vi "XY Graph Remove Head Outliers.vi"(8 "Error In":errorcluster, 9 "Peak Index (-1: unknown)":i32=-1, 11 "Plot in":cluster{"t Array":dbl[], "Array":dbl[]}) -> (0 "Error Out":errorcluster, 1 "# Outliers":i32, 3 "Plot out":cluster{"t Array":dbl[], "Array":dbl[]})   [LabVIEW 2021, in "XY Graph Add-Ons.lvlib"]
uses:
  XY Graph Add-Ons.lvlib
  <vilib>/gmath/statdist.llb/Normal Random.vi
  <vilib>/Analysis/NI_AALBase.lvlib
  <vilib>/gmath/NI_Gmath.lvlib
panel:
  # "see the License on the block diagram (Ctrl+E or Window:Show Block Diagram)"
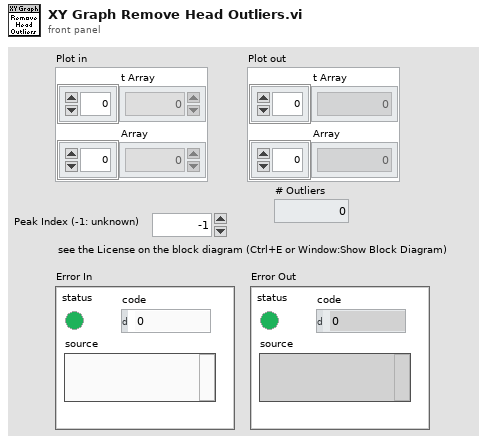
[diagram p1: front panel]
types:
  T1 = enum16{"Clipping", "Noisy Replacement", "Smoothing"}
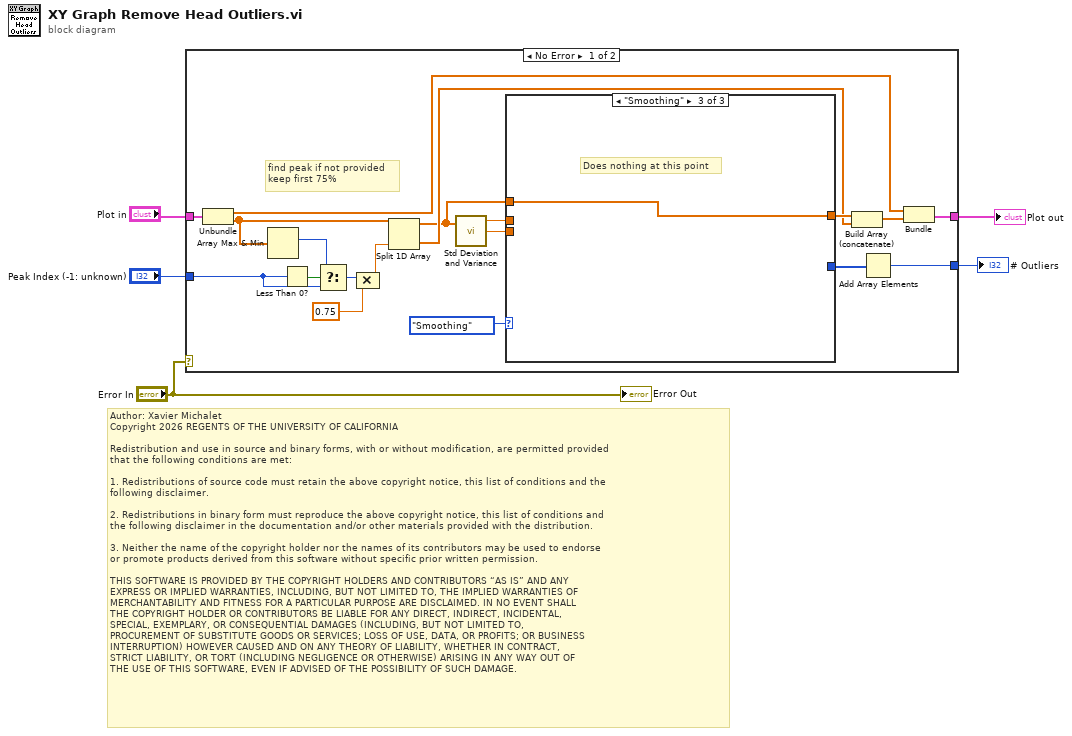
[diagram p0: block diagram]
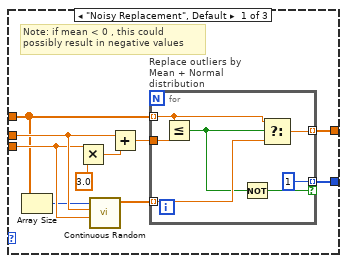
[diagram p2: hidden frame]
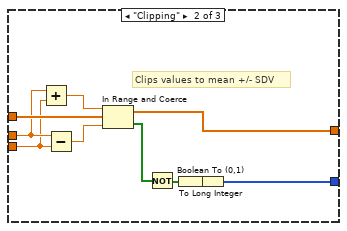
[diagram p3: hidden frame]
diagram:
  # "Author: Xavier Michalet\nCopyright 2026 REGENTS OF THE UNIVERSITY OF CALIFORNIA\n\nRedistribution and use in source and binary forms, with or without modification, are permitted provided\nthat the following conditions are met:\n\n1. Redistributions of source code must retain the above copyright notice, this list of conditions and the\nfollowing disclaimer.\n\n2. Redistributions in binary form must reproduce the above copyright notice, this list of conditions and\nthe following disclaimer in the documentation and/or other materials provided with the distribution.\n\n3. Neither the name of the copyright holder nor the names of its contributors may be used to endorse \nor promote products derived from this software without specific prior written permission.\n\nTHIS SOFTWARE IS PROVIDED BY THE COPYRIGHT HOLDERS AND CONTRIBUTORS “AS IS” AND ANY \nEXPRESS OR IMPLIED WARRANTIES, INCLUDING, BUT NOT LIMITED TO, THE IMPLIED WARRANTIES OF\nMERCHANTABILITY AND FITNESS FOR A PARTICULAR PURPOSE ARE DISCLAIMED. IN NO EVENT SHALL\nTHE COPYRIGHT HOLDER OR CONTRIBUTORS BE LIABLE FOR ANY DIRECT, INDIRECT, INCIDENTAL, \nSPECIAL, EXEMPLARY, OR CONSEQUENTIAL DAMAGES (INCLUDING, BUT NOT LIMITED TO, \nPROCUREMENT OF SUBSTITUTE GOODS OR SERVICES; LOSS OF USE, DATA, OR PROFITS; OR BUSINESS\nINTERRUPTION) HOWEVER CAUSED AND ON ANY THEORY OF LIABILITY, WHETHER IN CONTRACT, \nSTRICT LIABILITY, OR TORT (INCLUDING NEGLIGENCE OR OTHERWISE) ARISING IN ANY WAY OUT OF\nTHE USE OF THIS SOFTWARE, EVEN IF ADVISED OF THE POSSIBILITY OF SUCH DAMAGE."
  n1 = case shown="No Error" "Error In" {
    tunnel: "Plot in" -> [w20 w53]
    tunnel: "Peak Index (-1: unknown)" -> [w19 _]
    tunnel: [w10 w53] -> w3
    tunnel: [w8 _] -> w2
    frame No Error {
      # "find peak if not provided\nkeep first 75%"
      n2 = Unbundle(w20) -> ("t Array"=w11:dbl[], "Array"=w22:dbl[])
      n3 = Array Max & Min(array=w22) -> (max index (indices)=w21:i32)  [unwired: 3 out]
      n4 = Less Than 0?(x=w19) -> (x < 0?=w24:bool)
      n5 = Select(t=w21, s=w24, f=w19) -> (s? t:f=w23:i32)
      n6 = Compound Arithmetic op=MULTIPLY(w23, 0.75 ("value")) -> (w18:dbl)
      n7 = Split 1D Array(array=w22, index=w18) -> (first subarray=w7:dbl[], second subarray=w13:dbl[])
      n8 = call <vilib>:"Std Deviation and Variance.vi"("X"=w7) -> ("mean"=w16:dbl, "standard deviation"=w15:dbl)  [unwired: 1 in, 1 out]
      n9 = case shown="\"Smoothing\"" T1."Smoothing" {
        tunnel: w16 -> [w31 w49 _]
        tunnel: w15 -> [w30 w48 _]
        tunnel: w7 -> [w25 w51 w52]
        tunnel: [w28 w46 w52] -> w14
        tunnel: [w27 w42 _] -> w9
        frame "Noisy Replacement", Default {
          # "Note: if mean < 0 , this could possibly result in negative values"
          n10 = Array Size(array=w25) -> (size(s)=w26:i32)
          n11 = Multiply(x=w30, y=3.0) -> (x*y=w33:dbl)
          n12 = call-poly <vilib>:"Continuous Random.vi"("std"=w30, "mean"=w31, "samples"=w26) -> ("normal random data"=w29:dbl[])  [unwired: 7 in, 1 out]
          n13 = Add(x=w31, y=w33) -> (x+y=w32:dbl)
          n14 = for "Replace outliers by Mean + Normal distribution" {
            tunnel: w25 -> [w40] mode=indexing
            tunnel: w32 -> [w41]
            tunnel: [w39] -> w28 mode=indexing
            tunnel: w29 -> [w38] mode=indexing
            tunnel: [1] -> w27 mode=indexing if=w35
            n15 = Less Or Equal?(x=w40, y=w41) -> (x <= y?=w36:bool)
            n16 = Not(x=w36) -> (.not. x?=w35:bool)
            n17 = Select(t=w40, s=w36, f=w38) -> (s? t:f=w39:dbl)
          }
        }
        frame "Clipping" {
          # "Clips values to mean +/- SDV"
          n18 = Add(x=w49, y=w48) -> (x+y=w50:dbl)
          n19 = Subtract(x=w49, y=w48) -> (x-y=w47:dbl)
          n20 = In Range and Coerce(upper limit=w50, x=w51, lower limit=w47) -> (coerced(x)=w46:dbl[], In Range?=w45:bool[])
          n21 = Not(x=w45) -> (.not. x?=w44:bool[])
          n22 = Boolean To (0,1)(Boolean=w44) -> (0, 1=w43:i16[])
          n23 = To Long Integer(number=w43) -> (32bit integer=w42:i32[])
        }
        frame "Smoothing" {
          # "Does nothing at this point"
        }
      }
      n24 = Build Array (concatenate)(w14, w13) -> (w12:dbl[])
      n25 = Add Array Elements(numeric array=w9) -> (sum=w8:i32)
      n26 = Bundle("t Array"=w11, w12) -> (w10:cluster{"t Array":dbl[], dbl[]})  [unwired: 1 in]
    }
    frame Error {
    }
  }
  "Plot out" <- w3
  "# Outliers" <- w2
  "Error Out" <- "Error In"
